vi "DSC TSV Date Time to Timestamp.vi"(8 "error in":errorcluster, 11 "all rows":string[][](array[string])) -> (0 "error out":errorcluster, 2 "Timestamps":timestamp[](array[timestamp]), 3 "array of clusters":cluster{"String":string}[](array[cluster]))   [LabVIEW 2019, in "LV-Data.PGSQL.lvclass"]
uses:
  LV-Data.PGSQL.lvclass
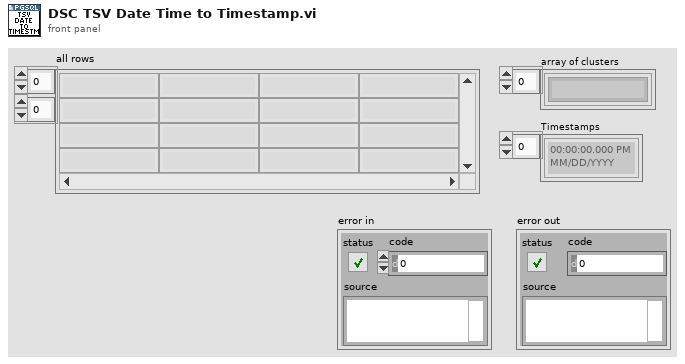
[diagram p1: front panel]
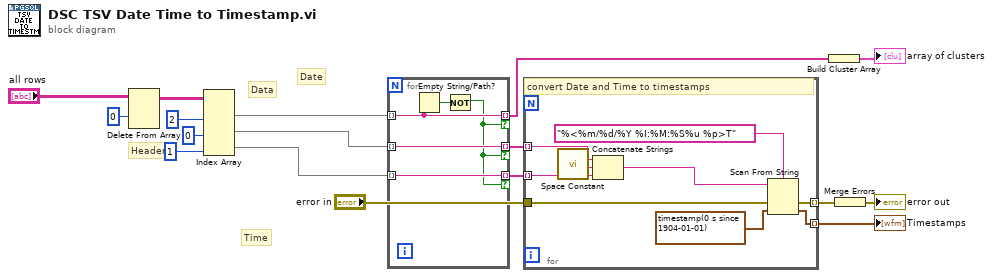
[diagram p0: block diagram]
diagram:
  # "Data"
  # "Time"
  # "Date"
  # "Header"
  n1 = Delete From Array(array="all rows", index (row)=0) -> (array with subset deleted=w9:string[][])  [unwired: 2 in, 1 out]
  n2 = Index Array(array=w9, index (col) #1=2 ("disabled index (col)"), index (col) #2=0 ("disabled index (col)"), index (col) #3=1 ("disabled index (col)")) -> (element #1=w3:string[], element #2=w1:string[], element #3=w2:string[])  [unwired: 3 in]
  n3 = for {
    tunnel: w3 -> [w22] mode=indexing
    tunnel: [w22] -> w11 mode=indexing if=w18
    tunnel: [w20] -> w13 mode=indexing if=w18
    tunnel: w1 -> [w20] mode=indexing
    tunnel: [w19] -> w12 mode=indexing if=w18
    tunnel: w2 -> [w19] mode=indexing
    n4 = Empty String/Path?(string/path=w22) -> (empty?=w21:bool)
    n5 = Not(x=w21) -> (.not. x?=w18:bool)
  }
  n6 = for {
    tunnel: w13 -> [w28] mode=indexing
    tunnel: w12 -> [w27] mode=indexing
    tunnel: [w30] -> w17 mode=indexing
    tunnel: "error in" -> [w24]
    tunnel: [w23] -> w16 mode=indexing
    # "convert Date and Time to timestamps"
    n7 = call <vilib>:"Space Constant.vi"() -> ("String"=w25:string)
    n8 = Concatenate Strings(w28, w25, w27) -> (w26:string)
    n9 = Scan From String(format string="%<%m/%d/%Y %I:%M:%S%u %p>T", input string=w26, error in=w24, default 1=timestamp(0 s since 1904-01-01) ("default value 1")) -> (error out=w23:errorcluster, output 1=w30:timestamp)  [unwired: 1 in, 2 out]
  }
  "Timestamps" <- w17
  n10 = Build Cluster Array(w11) -> (→"array of clusters":cluster{"String":string}[])
  n11 = Merge Errors(w16) -> (→"error out":errorcluster)
